vi "Process Results File.vi"() -> ()   [LabVIEW 2019]
panel:
  out "File Match Count":i32
  out "Found Match Count":i32
  out "file matches adc":cluster{"Numeric":i32, "Numeric":i32}[](array[cluster])
  out "Matches (ADC only)":cluster{"ADC Value":i32, "ADC Value":i32}[](array[cluster])
  out "Matches":T1(array[cluster])
  out "min index(es)":i32
  out "min value":i32
  out "max index(es)":i32
  out "max value":i32
  out "Array":T2(array[cluster])
  out "Match Indices":T3(array[cluster])
  out "Unmatched 3-events":i32[](array[numeric])
  out "\"3-Events\" without a nearby match":i32
  out "Remaining \"3-Event\" count":i32
  out "size (no dups)":i32[](array[numeric])
  out "size (raw)":i32[](array[numeric])
  out "array (raw)":string[][](array[string])
  out "Array (no dups)":string[][](array[string])
  out "Duplicate 3 Events":i16
  in  "Path":path
  # "Recorded 427 coincident matches, with 485 \"3-events\"."
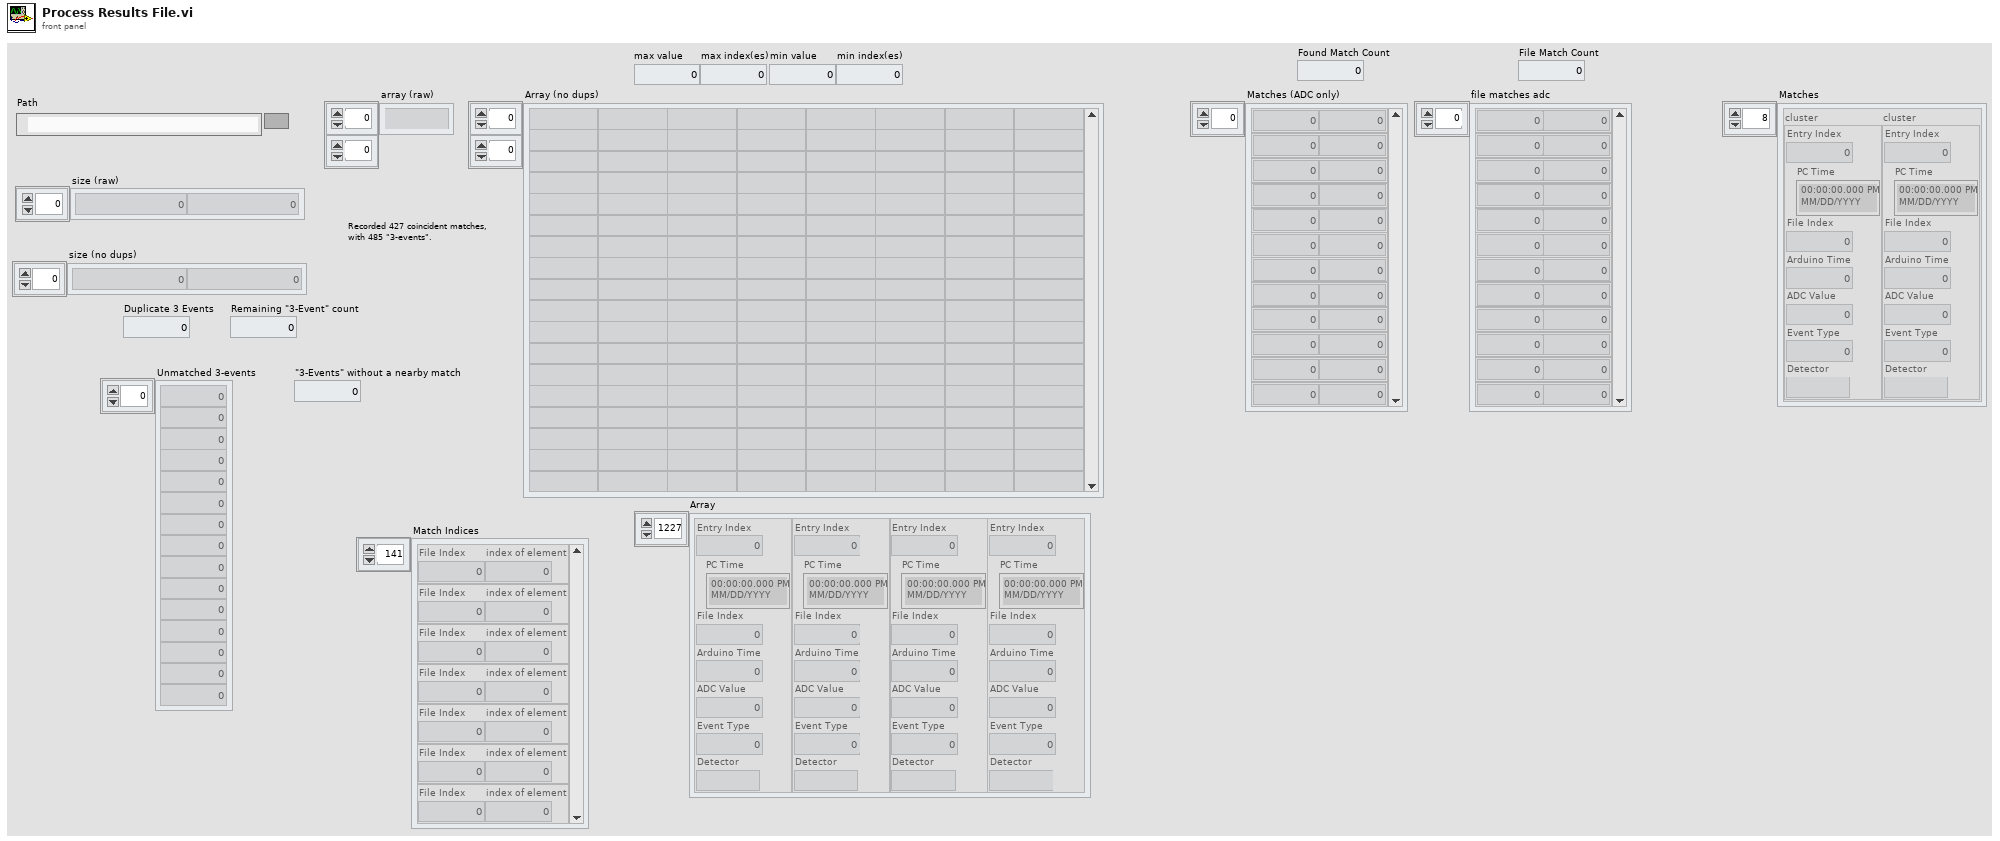
[diagram p1: front panel]
types:
  T1 = cluster{"cluster":cluster{"Entry Index":i32, "PC Time":timestamp, "File Index":i32, "Arduino Time":i32, "ADC Value":i32, "Event Type":i32, "Detector":string}, "cluster":cluster{"Entry Index":i32, "PC Time":timestamp, "File Index":i32, "Arduino Time":i32, "ADC Value":i32, "Event Type":i32, "Detector":string}}[]
  T2 = cluster{"Entry Index":i32, "PC Time":timestamp, "File Index":i32, "Arduino Time":i32, "ADC Value":i32, "Event Type":i32, "Detector":string}[]
  T3 = cluster{"File Index":i32, "index of element":i32}[]
  T4 = cluster{"Entry Index":i32, "PC Time":timestamp, "File Index":i32, "Arduino Time":i32, "ADC Value":i32, "Event Type":i32, "Detector":string}
  T5 = cluster{"cluster":cluster{"Entry Index":i32, "PC Time":timestamp, "File Index":i32, "Arduino Time":i32, "ADC Value":i32, "Event Type":i32, "Detector":string}, "cluster":cluster{"Entry Index":i32, "PC Time":timestamp, "File Index":i32, "Arduino Time":i32, "ADC Value":i32, "Event Type":i32, "Detector":string}}
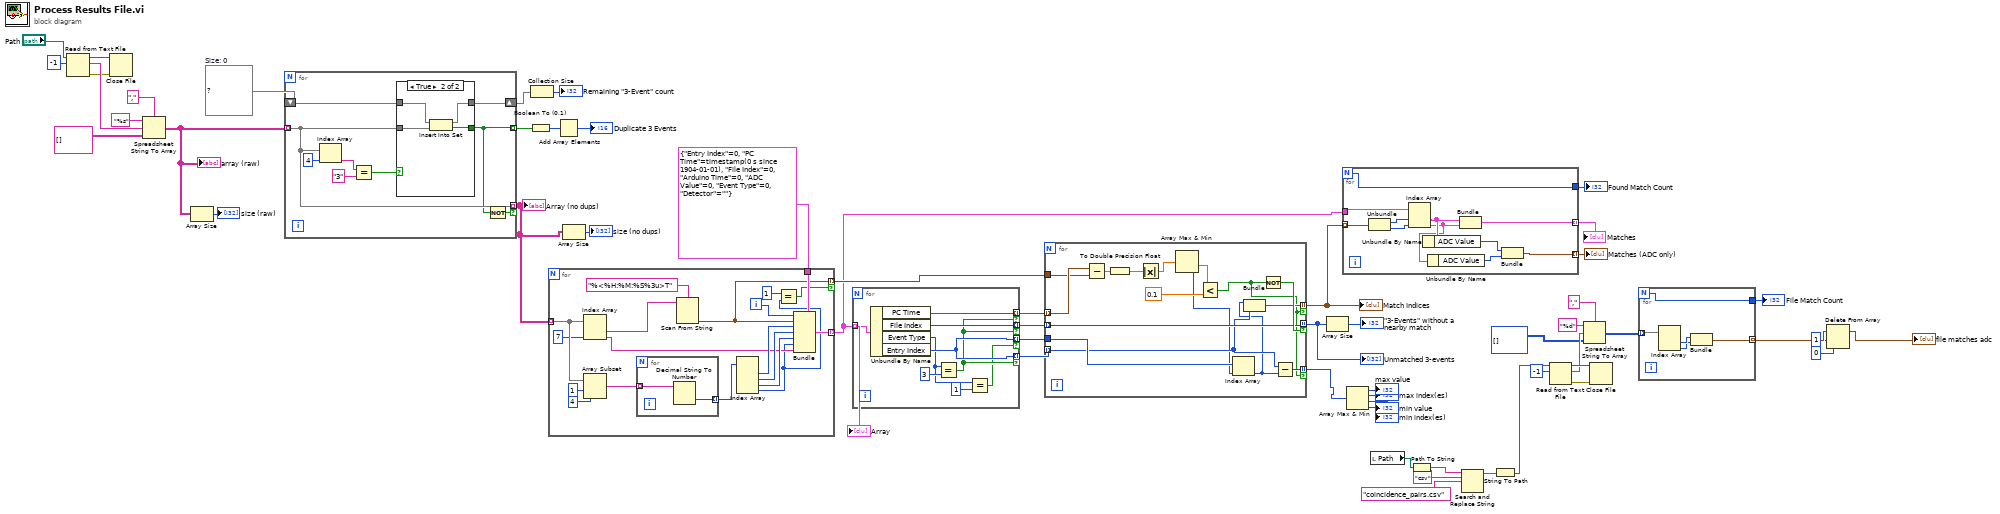
[diagram p0: block diagram]
diagram:
  w48 = set{string[]} {}  # Size: 0
  n1 = Read from Text File(file (use dialog)="Path", count=-1) -> (refnum out=w52:refnum<file>, text=w53:string, error out=w51:errorcluster)  [unwired: 2 in, 1 out]
  n2 = Close File(refnum=w52, error in=w51) -> ()  [unwired: 2 out]
  n3 = Spreadsheet String To Array(delimiter (Tab)=",", format string="%s", spreadsheet string=w53, array type (2D Dbl)=string[][] []) -> (array=w43:string[][])
  "array (raw)" <- w43
  n4 = Array Size(array=w43) -> (size(s)=→"size (raw)":i32[])
  n5 = for {
    tunnel: w43 -> [w58] mode=indexing
    shift-right: [w59] -> w40
    shift-left: w48 -> [w60]
    tunnel: [w57] -> w47 mode=indexing
    tunnel: [w58] -> w38 mode=indexing if=w56
    n6 = Index Array(array=w58, index=4) -> (element=w63:string)
    n7 = Equal?(x=w63, y="3") -> (x = y?=w61:bool)
    n8 = case shown="True" w61 {
      tunnel: w58 -> [_ w69]
      tunnel: w60 -> [w65 w68]
      tunnel: [w65 w67] -> w59
      tunnel: [_ w66] -> w57
      frame False {
      }
      frame True {
        n9 = Insert Into Set(10:w69, 11:w68) -> (2:w66:bool, 3:w67:set{string[]})
      }
    }
    n10 = Not(x=w57) -> (.not. x?=w56:bool)
  }
  "Array (no dups)" <- w38
  n11 = Boolean To (0,1)(Boolean=w47) -> (0, 1=w46:i16[])
  n12 = Collection Size(1:w40) -> (0:→"Remaining \"3-Event\" count":i32)
  n13 = for {
    tunnel: w38 -> [w85] mode=indexing
    tunnel: [w75] -> w23 mode=indexing
    tunnel: T4 {"Entry Index"=0, "PC Time"=timestamp(0 s since 1904-01-01), "File Index"=0, "Arduino Time"=0, "ADC Value"=0, "Event Type"=0, "Detector"=""} ("cluster") -> [w74]
    tunnel: [w73] -> w35 mode=indexing if=w71
    i -> [w86]
    n14 = Index Array(array=w85, index #2=7 ("index")) -> (element #1=w88:string, element #2=w77:string)  [unwired: 1 in]
    n15 = Array Subset(array=w85, index=1, length=4) -> (w82:string[])
    n16 = for {
      tunnel: w82 -> [w89] mode=indexing
      tunnel: [w90] -> w81 mode=indexing
      n17 = Decimal String To Number(string=w89) -> (number=w90:i32)  [unwired: 2 in, 1 out]
    }
    n18 = Scan From String(format string="%<%H:%M:%S%3u>T", input string=w88) -> (output 1=w73:timestamp)  [unwired: 3 in, 3 out]
    n19 = Index Array(array=w81) -> (element #1=w80:i32, element #2=w79:i32, element #3=w78:i32, element #4=w72:i32)  [unwired: 4 in]
    n20 = Equal?(x=1, y=w72) -> (x = y?=w71:bool)
    n21 = Bundle(cluster=w74, "Entry Index"=w86, "PC Time"=w73, "File Index"=w80, "Arduino Time"=w79, "ADC Value"=w78, "Event Type"=w72, "Detector"=w77) -> (w75:T4)
  }
  "Array" <- w23
  n22 = Add Array Elements(numeric array=w46) -> (sum=→"Duplicate 3 Events":i16)
  n23 = Array Size(array=w38) -> (size(s)=→"size (no dups)":i32[])
  n24 = for {
    tunnel: w23 -> [w99] mode=indexing
    tunnel: [w98] -> w36 mode=indexing if=w94
    tunnel: [w96] -> w32 mode=indexing if=w94
    tunnel: [w95] -> w31 mode=indexing if=w94
    tunnel: [w95] -> w30 mode=indexing if=w91
    n25 = Unbundle By Name(w99) -> ("PC Time"=w98:timestamp, "File Index"=w96:i32, "Event Type"=w93:i32, "Entry Index"=w95:i32)
    n26 = Equal?(x=w93, y=3) -> (x = y?=w94:bool)
    n27 = Equal?(x=w93, y=1) -> (x = y?=w91:bool)
  }
  n28 = for {
    tunnel: w36 -> [w114] mode=indexing
    tunnel: w35 -> [w113]
    tunnel: w32 -> [w109] mode=indexing
    tunnel: [w109] -> w34 mode=indexing if=w115
    tunnel: [w108] -> w24 mode=indexing if=w100
    tunnel: w31 -> [w105] mode=indexing
    tunnel: w30 -> [w107]
    tunnel: [w106] -> w29 mode=indexing if=w100
    n29 = Subtract(x=w114, y=w113) -> (x-y=w112:dbl[])
    n30 = To Double Precision Float(number=w112) -> (double precision float=w111:dbl[])
    n31 = Absolute Value(x=w111) -> (abs(x)=w103:dbl[])
    n32 = Array Max & Min(array=w103) -> (min value=w102:dbl, min index (indices)=w101:i32)  [unwired: 2 out]
    n33 = Less?(x=w102, y=0.1) -> (x < y?=w100:bool)
    n34 = Index Array(array=w107, index=w101) -> (element=w104:i32)
    n35 = Bundle("Entry Index"=w104, "Entry Index"=w105) -> (w108:cluster{"Entry Index":i32, "Entry Index":i32})  [unwired: 1 in]
    n36 = Not(x=w100) -> (.not. x?=w115:bool)
    n37 = Subtract(x=w105, y=w104) -> (x-y=w106:i32)
  }
  "Unmatched 3-events" <- w34
  "Match Indices" <- w24
  n38 = Array Size(array=w34) -> (size(s)=→"\"3-Events\" without a nearby match":i32)
  n39 = for {
    N -> [w116]
    tunnel: w24 -> [w126] mode=indexing
    tunnel: w23 -> [w124]
    tunnel: [w122] -> w22 mode=indexing
    tunnel: [w117] -> w21 mode=indexing
    tunnel: [w116] -> w2
    n40 = Unbundle(w126) -> ("Entry Index"=w125:i32, "Entry Index"=w123:i32)
    n41 = Index Array(array=w124, index #1=w125, index #2=w123) -> (element #1=w121:T4, element #2=w120:T4)
    n42 = Unbundle By Name(w121) -> ("ADC Value"=w119:i32)
    n43 = Unbundle By Name(w120) -> ("ADC Value"=w118:i32)
    n44 = Bundle("cluster"=w121, "cluster"=w120) -> (w122:T5)  [unwired: 1 in]
    n45 = Bundle("ADC Value"=w119, "ADC Value"=w118) -> (w117:cluster{"ADC Value":i32, "ADC Value":i32})  [unwired: 1 in]
  }
  "Matches" <- w22
  "Matches (ADC only)" <- w21
  "Found Match Count" <- w2
  n46 = Array Max & Min(array=w29) -> (max value=→"max value":i32, max index (indices)=→"max index(es)":i32, min value=→"min value":i32, min index (indices)=→"min index(es)":i32)
  n47 = local read "Path"() -> (w17:path)
  n48 = Path To String(path=w17) -> (string=w18:string)
  n49 = Search and Replace String(input string=w18, search string="csv", replace string="coincidence_pairs.csv" ("replace string (\"\")")) -> (result string=w14:string)  [unwired: 5 in, 3 out]
  n50 = String To Path(string=w14) -> (path=w13:path)
  n51 = Read from Text File(file (use dialog)=w13, count=-1) -> (refnum out=w20:refnum<file>, text=w11:string, error out=w19:errorcluster)  [unwired: 2 in, 1 out]
  n52 = Spreadsheet String To Array(delimiter (Tab)=",", format string="%d", spreadsheet string=w11, array type (2D Dbl)=i32[][] []) -> (array=w7:i32[][])
  n53 = Close File(refnum=w20, error in=w19) -> ()  [unwired: 2 out]
  n54 = for {
    N -> [w127]
    tunnel: w7 -> [w131] mode=indexing
    tunnel: [w128] -> w6 mode=indexing
    tunnel: [w127] -> w1
    n55 = Index Array(array=w131) -> (element #1=w130:i32, element #2=w129:i32)  [unwired: 2 in]
    n56 = Bundle(w130, w129) -> (w128:cluster{i32, i32})  [unwired: 1 in]
  }
  "File Match Count" <- w1
  n57 = Delete From Array(array=w6, length=1, index=0) -> (array with subset deleted=→"file matches adc":cluster{i32, i32}[])  [unwired: 1 out]
